vi "ComStrView.vi"(6 "StrInit":string, 7 "Hex？":bool, 8 "error in":errorcluster caption="错误输入（无错误）", 9 "ComConn":refnum<vi>, 10 "ReactStrIn":string, 11 "CMDIn":string) -> (0 "error out":errorcluster caption="错误输出", 3 "连接字符串显示":string)   [LabVIEW 2013]
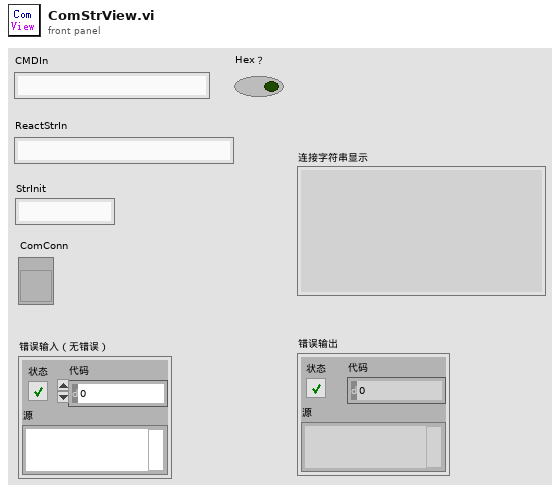
[diagram p1: front panel]
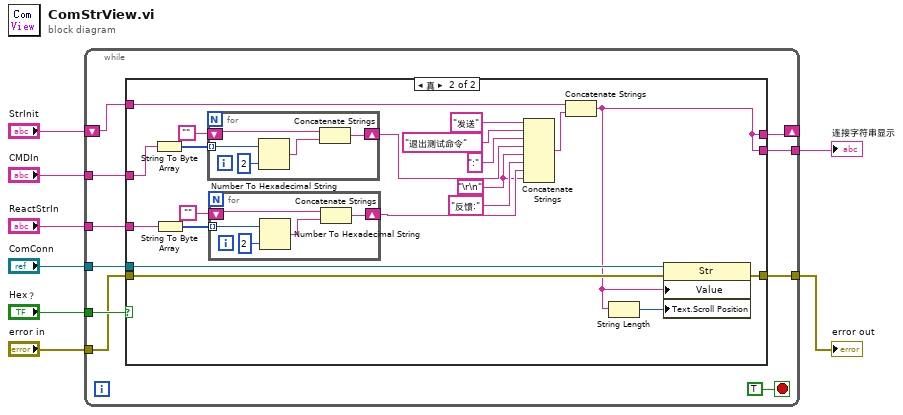
[diagram p0: block diagram]
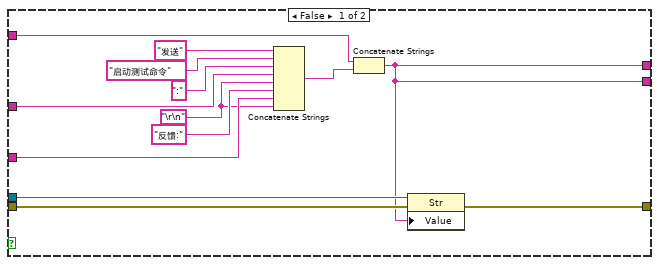
[diagram p2: hidden frame]
diagram:
  n1 = while {
    tunnel: "Hex？" -> [w18]
    tunnel: "CMDIn" -> [w17]
    tunnel: "ComConn" -> [w16]
    tunnel: "ReactStrIn" -> [w15]
    tunnel: "error in" -> [w14]
    tunnel: [w13] -> w3
    tunnel: [w12] -> w2
    shift-right: [w10] -> _
    shift-left: "StrInit" -> [w9]
    stop <- TRUE stop-if-true
    n2 = case shown="真" w18 {
      tunnel: w17 -> [w28 w51]
      tunnel: w16 -> [w24 w38]
      tunnel: w15 -> [w26 w46]
      tunnel: w14 -> [w23 w37]
      tunnel: [w22 w36] -> w13
      tunnel: [w19 w32] -> w12
      tunnel: [w19 w32] -> w10
      tunnel: w9 -> [w20 w34]
      frame False {
        w25 = "\r\n"
        n3 = Concatenate Strings("发送", "启动测试命令", ":", w28, w25, "反馈:", w26, w25) -> (w21:string)
        n4 = Concatenate Strings(w20, w21) -> (w19:string)
        n5 = property class="Str"(reference=w24, error in=w23, "Value"=w19) -> (error out=w22:errorcluster)  [unwired: 1 out]
      }
      frame True {
        w39 = "\r\n"
        n6 = String To Byte Array(string=w51) -> (unsigned byte array=w50:u8[])
        n7 = String To Byte Array(string=w46) -> (unsigned byte array=w47:u8[])
        n8 = for {
          tunnel: w50 -> [w60] mode=indexing
          shift-right: [w59] -> w42
          shift-left: "" -> [w58]
          n9 = Number To Hexadecimal String(1:2, 2:w60) -> (0:w57:string)
          n10 = Concatenate Strings(w58, w57) -> (w59:string)
        }
        n11 = for {
          tunnel: w47 -> [w55] mode=indexing
          shift-right: [w54] -> w40
          shift-left: "" -> [w53]
          n12 = Number To Hexadecimal String(1:2, 2:w55) -> (0:w52:string)
          n13 = Concatenate Strings(w53, w52) -> (w54:string)
        }
        n14 = Concatenate Strings("发送", "退出测试命令", ":", w42, w39, "反馈:", w40, w39) -> (w35:string)
        n15 = Concatenate Strings(w34, w35) -> (w32:string)
        n16 = String Length(string=w32) -> (length=w33:i32)
        n17 = property class="Str"(reference=w38, error in=w37, "Value"=w32, "Text.Scroll Position"=w33) -> (error out=w36:errorcluster)  [unwired: 1 out]
      }
    }
  }
  "error out" <- w3
  "连接字符串显示" <- w2
